vi "WT1600 Multicard Total Current.vi"(0 "WT1600":refnum<visa-resource-name>, 5 "error in (no error)":errorcluster) -> (14 "dup VISA session":refnum<visa-resource-name>, 15 "Total Current":dbl, 16 "i1":dbl, 17 "i 2":dbl, 18 "I3":dbl, 19 "error out":errorcluster)   [LabVIEW 2012]
panel:
  out "Read Strings":string
  out "Measure":dbl[](array[numeric]) format="%^.4e"
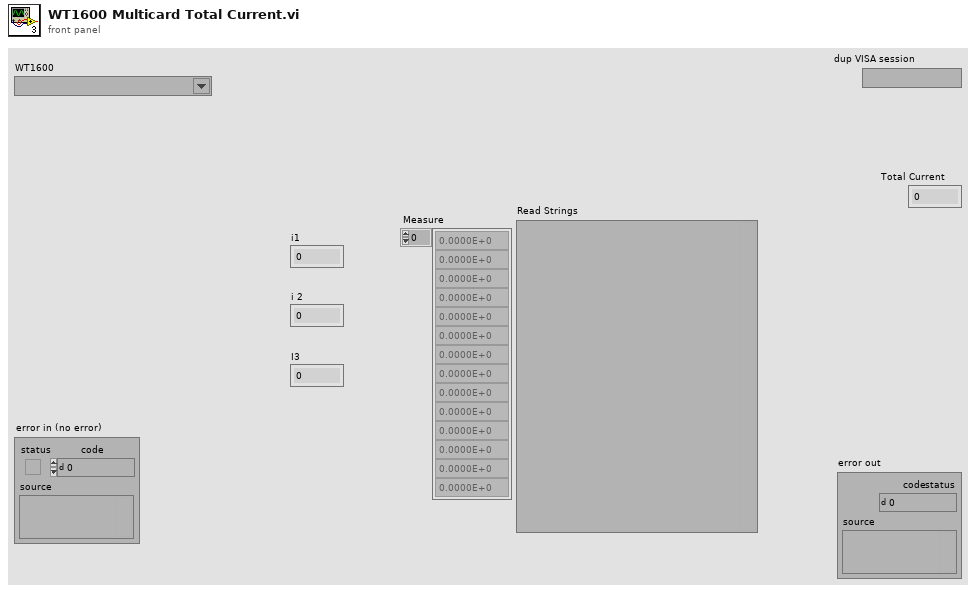
[diagram p1: front panel]
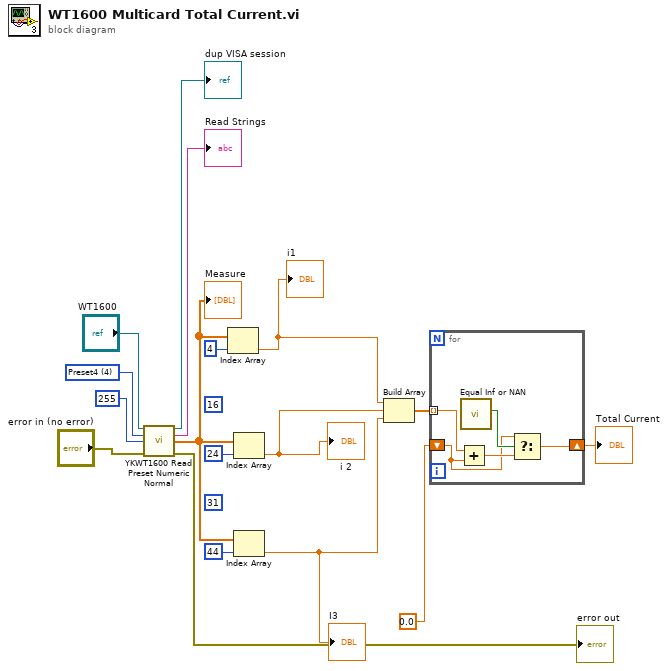
[diagram p0: block diagram]
diagram:
  (unwired) 31 ("index")
  (unwired) 16 ("index")
  w13 = u16 4 items=["", "Preset1", "Preset2", "Preset3", "Preset4"] ("Preset (2: Preset 2)")
  n1 = call <instrlib>:"YKWT1600 Read Preset Numeric Normal.vi"("VISA session"="WT1600", "Preset (2: Preset 2)"=w13, "Number of Item (15)"=u16 255, "error in (no error)"="error in (no error)") -> ("dup VISA session"=→"dup VISA session":refnum<visa-resource-name>, "Read Strings"=→"Read Strings":string, "Measure"=w10:dbl[], "error out"=→"error out":errorcluster)  [unwired: 8 in]
  "Measure" <- w10
  n2 = Index Array(array=w10, index=4) -> (element=w3:dbl)
  "i1" <- w3
  n3 = Index Array(array=w10, index=24) -> (element=w2:dbl)
  "i 2" <- w2
  n4 = Index Array(array=w10, index=44) -> (element=w1:dbl)
  "I3" <- w1
  n5 = Build Array(w3, w2, w1) -> (w6:dbl[])
  n6 = for {
    tunnel: w6 -> [w18] mode=indexing
    shift-right: [w21] -> w4
    shift-left: 0.0 -> [w19]
    n7 = Add(x=w18, y=w19) -> (x+y=w20:dbl)
    n8 = call "Equal Inf or NAN.vi"() -> ("NaN or Inf"=w22:bool)  [unwired: 11 in]
    n9 = Select(t=w19, s=w22, f=w20) -> (s? t:f=w21:dbl)
  }
  "Total Current" <- w4
